vi "roundcreate.vi"(1 "D":cluster{dbl, dbl}, 2 "C":cluster{dbl, dbl}, 3 "B":cluster{dbl, dbl}, 4 "A":cluster{dbl, dbl}) -> (0 "Array":cluster{dbl, dbl}[](array[cluster]))   [LabVIEW 2019]
panel:
  out "XY Graph":cluster{cluster{dbl, dbl}[]}[](graph)
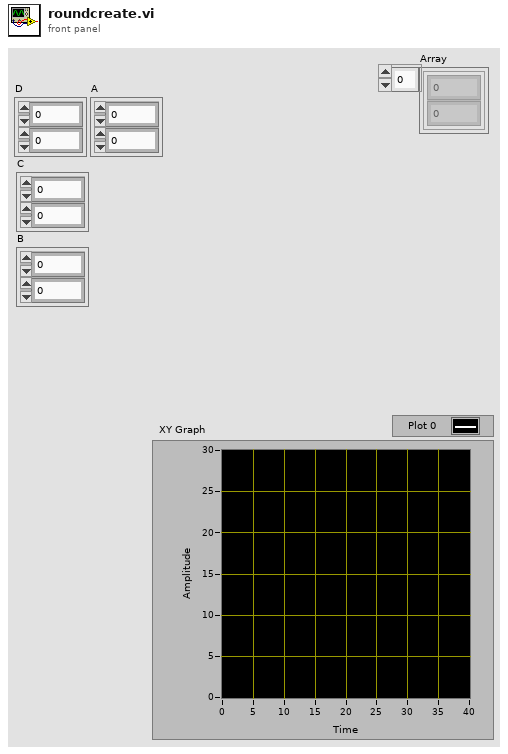
[diagram p1: front panel]
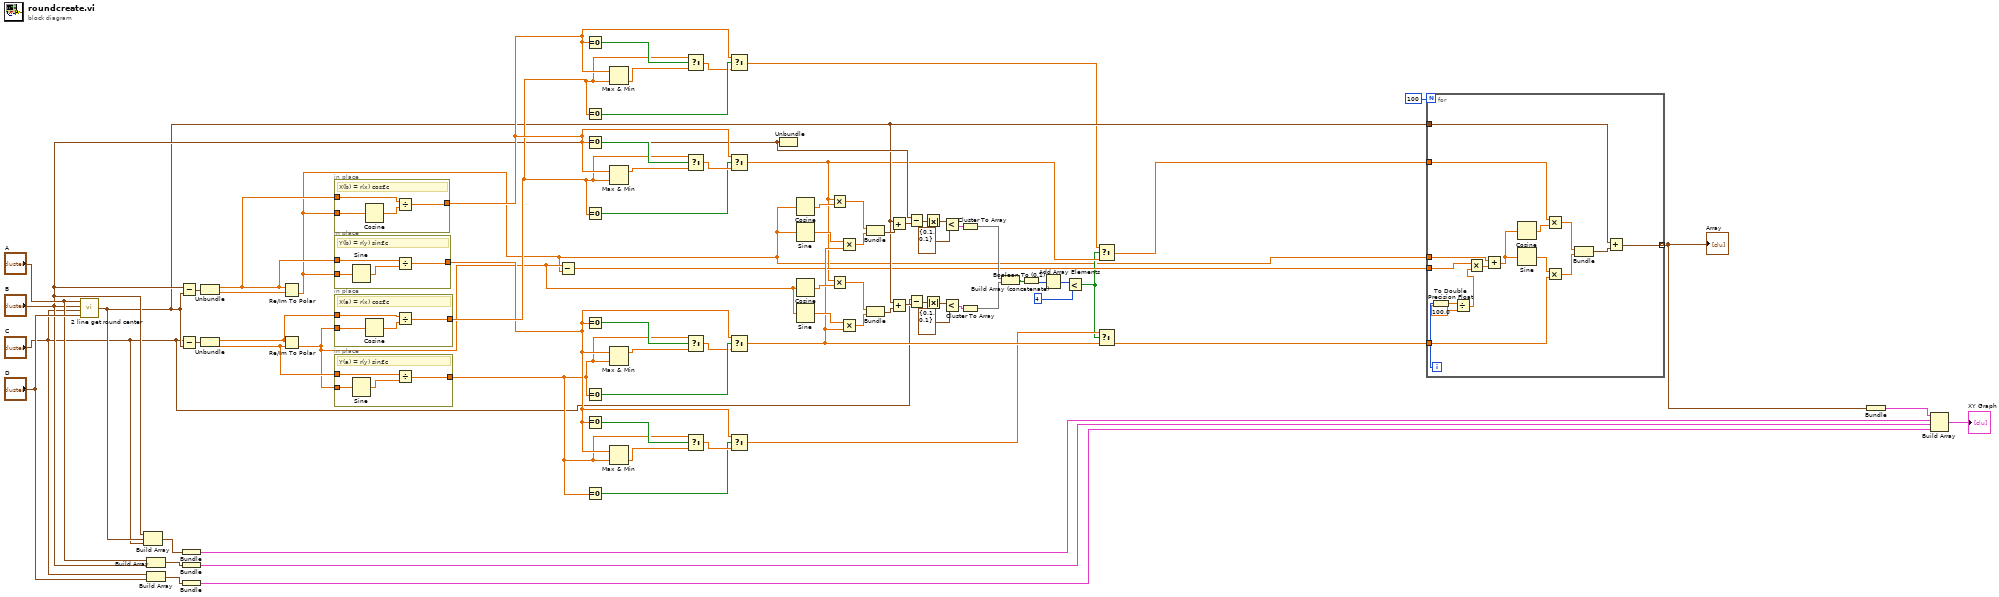
[diagram p0: block diagram]
diagram:
  n1 = call "2 line get round center.vi"("D"="D", "C"="C", "B"="B", "A"="A") -> ("round center"=w18:cluster{dbl, dbl})
  n2 = Build Array("B", w18, "C") -> (w74:cluster{dbl, dbl}[])
  n3 = Build Array("A", "B") -> (w73:cluster{dbl, dbl}[])
  n4 = Build Array("C", "D") -> (w72:cluster{dbl, dbl}[])
  n5 = Subtract(x="B", y=w18) -> (x-y=w76:cluster{dbl, dbl})
  n6 = Subtract(x="C", y=w18) -> (x-y=w77:cluster{dbl, dbl})
  n7 = Bundle(w74) -> (w70:cluster{cluster{dbl, dbl}[]})  [unwired: 1 in]
  n8 = Bundle(w73) -> (w69:cluster{cluster{dbl, dbl}[]})  [unwired: 1 in]
  n9 = Bundle(w72) -> (w68:cluster{cluster{dbl, dbl}[]})  [unwired: 1 in]
  n10 = Unbundle(w76) -> (w40:dbl, w41:dbl)
  n11 = Unbundle(w77) -> (w67:dbl, w66:dbl)
  n12 = Re/Im To Polar(2:w41, 3:w40) -> (0:w1:dbl)  [unwired: 1 out]
  n13 = Re/Im To Polar(2:w66, 3:w67) -> (0:w19:dbl)  [unwired: 1 out]
  n14 = in-place {
    in-place-border: w40 -> [w80]
    in-place-border: w1 -> [w81]
    in-place-border: [w78] -> w52
    # "X(b) = r(x) cos£c"
    n15 = Cosine(x=w81) -> (cos(x)=w79:dbl)
    n16 = Divide(x=w80, y=w79) -> (x/y=w78:dbl)
  }
  n17 = in-place {
    in-place-border: w1 -> [w84]
    in-place-border: w40 -> [w83]
    in-place-border: [w82] -> w46
    # "Y(b) = r(y) sin£c"
    n18 = Sine(x=w84) -> (sin(x)=w85:dbl)
    n19 = Divide(x=w83, y=w85) -> (x/y=w82:dbl)
  }
  n20 = in-place {
    in-place-border: w19 -> [w88]
    in-place-border: w67 -> [w87]
    in-place-border: [w86] -> w51
    # "X(a) = r(x) cos£c"
    n21 = Cosine(x=w88) -> (cos(x)=w89:dbl)
    n22 = Divide(x=w87, y=w89) -> (x/y=w86:dbl)
  }
  n23 = in-place {
    in-place-border: w66 -> [w92]
    in-place-border: w19 -> [w91]
    in-place-border: [w90] -> w45
    # "Y(a) = r(y) sin£c"
    n24 = Sine(x=w91) -> (sin(x)=w93:dbl)
    n25 = Divide(x=w92, y=w93) -> (x/y=w90:dbl)
  }
  n26 = Subtract(x=w19, y=w1) -> (x-y=w6:dbl)
  n27 = Equal To 0?(x=w52) -> (x = 0?=w53:bool)
  n28 = Equal To 0?(x=w51) -> (x = 0?=w55:bool)
  n29 = Equal To 0?(x=w52) -> (x = 0?=w65:bool)
  n30 = Equal To 0?(x=w51) -> (x = 0?=w63:bool)
  n31 = Equal To 0?(x=w46) -> (x = 0?=w60:bool)
  n32 = Equal To 0?(x=w45) -> (x = 0?=w62:bool)
  n33 = Equal To 0?(x=w46) -> (x = 0?=w49:bool)
  n34 = Equal To 0?(x=w45) -> (x = 0?=w47:bool)
  n35 = Max & Min(x=w52, y=w51) -> (min(x,y)=w56:dbl)  [unwired: 1 out]
  n36 = Max & Min(x=w52, y=w51) -> (max(x,y)=w35:dbl)  [unwired: 1 out]
  n37 = Max & Min(x=w46, y=w45) -> (max(x,y)=w36:dbl)  [unwired: 1 out]
  n38 = Max & Min(x=w46, y=w45) -> (min(x,y)=w50:dbl)  [unwired: 1 out]
  n39 = Select(t=w51, s=w53, f=w56) -> (s? t:f=w54:dbl)
  n40 = Select(t=w51, s=w65, f=w35) -> (s? t:f=w64:dbl)
  n41 = Select(t=w45, s=w60, f=w36) -> (s? t:f=w61:dbl)
  n42 = Select(t=w45, s=w49, f=w50) -> (s? t:f=w48:dbl)
  n43 = Select(t=w52, s=w55, f=w54) -> (s? t:f=w5:dbl)
  n44 = Select(t=w52, s=w63, f=w64) -> (s? t:f=w4:dbl)
  n45 = Select(t=w46, s=w62, f=w61) -> (s? t:f=w20:dbl)
  n46 = Select(t=w46, s=w47, f=w48) -> (s? t:f=w7:dbl)
  n47 = Unbundle("B") -> ()  [unwired: 2 out]
  n48 = Cosine(x=w1) -> (cos(x)=w44:dbl)
  n49 = Sine(x=w1) -> (sin(x)=w43:dbl)
  n50 = Cosine(x=w19) -> (cos(x)=w21:dbl)
  n51 = Sine(x=w19) -> (sin(x)=w22:dbl)
  n52 = Multiply(x=w4, y=w44) -> (x*y=w39:dbl)
  n53 = Multiply(x=w4, y=w21) -> (x*y=w23:dbl)
  n54 = Multiply(x=w43, y=w20) -> (x*y=w38:dbl)
  n55 = Multiply(x=w22, y=w20) -> (x*y=w24:dbl)
  n56 = Bundle(w39, w38) -> (w37:cluster{dbl, dbl})  [unwired: 1 in]
  n57 = Bundle(w23, w24) -> (w25:cluster{dbl, dbl})  [unwired: 1 in]
  n58 = Add(x=w18, y=w37) -> (x+y=w34:cluster{dbl, dbl})
  n59 = Add(x=w18, y=w25) -> (x+y=w26:cluster{dbl, dbl})
  n60 = Subtract(x="B", y=w34) -> (x-y=w32:cluster{dbl, dbl})
  n61 = Subtract(x="C", y=w26) -> (x-y=w27:cluster{dbl, dbl})
  n62 = Absolute Value(x=w32) -> (abs(x)=w31:cluster{dbl, dbl})
  n63 = Absolute Value(x=w27) -> (abs(x)=w28:cluster{dbl, dbl})
  n64 = Less?(x=w31, y=cluster{dbl, dbl} {0.1, 0.1}) -> (x < y?=w16:cluster{bool, bool})
  n65 = Less?(x=w28, y=cluster{dbl, dbl} {0.1, 0.1}) -> (x < y?=w15:cluster{bool, bool})
  n66 = Cluster To Array(cluster=w16) -> (array=w14:bool[])
  n67 = Cluster To Array(cluster=w15) -> (array=w13:bool[])
  n68 = Build Array (concatenate)(w14, w13) -> (w12:bool[])
  n69 = Boolean To (0,1)(Boolean=w12) -> (0, 1=w11:i16[])
  n70 = Add Array Elements(numeric array=w11) -> (sum=w10:i16)
  n71 = Less?(x=w10, y=i16 4) -> (x < y?=w3:bool)
  n72 = Select(t=w5, s=w3, f=w4) -> (s? t:f=w2:dbl)
  n73 = Select(t=w7, s=w3, f=w20) -> (s? t:f=w8:dbl)
  n74 = for {
    N: 100 -> [_]
    tunnel: w6 -> [w107]
    tunnel: w1 -> [w104]
    tunnel: w2 -> [w101]
    tunnel: w8 -> [w99]
    tunnel: w18 -> [w95]
    tunnel: [w94] -> w58 mode=indexing
    i -> [w109]
    n75 = To Double Precision Float(number=w109) -> (double precision float=w110:dbl)
    n76 = Divide(x=w110, y=100.0) -> (x/y=w106:dbl)
    n77 = Multiply(x=w107, y=w106) -> (x*y=w105:dbl)
    n78 = Add(x=w104, y=w105) -> (x+y=w103:dbl)
    n79 = Cosine(x=w103) -> (cos(x)=w102:dbl)
    n80 = Sine(x=w103) -> (sin(x)=w100:dbl)
    n81 = Multiply(x=w101, y=w102) -> (x*y=w98:dbl)
    n82 = Multiply(x=w100, y=w99) -> (x*y=w97:dbl)
    n83 = Bundle(w98, w97) -> (w96:cluster{dbl, dbl})  [unwired: 1 in]
    n84 = Add(x=w95, y=w96) -> (x+y=w94:cluster{dbl, dbl})
  }
  "Array" <- w58
  n85 = Bundle(w58) -> (w57:cluster{cluster{dbl, dbl}[]})  [unwired: 1 in]
  n86 = Build Array(w57, w70, w69, w68) -> (→"XY Graph":cluster{cluster{dbl, dbl}[]}[])
